vi "keccak.ip.fifo.control.export.vi"(0 "Reset":bool, 1 "TS_RESULTS.Ready":bool, 2 "TS_PARMS.Element":u64, 3 "TS_PARMS.Valid":bool, 4 "TS_DATA.Element":u64, 5 "TS_DATA.Valid":bool) -> (14 "TS_RESULTS.Element":u64, 15 "TS_RESULTS.Valid":bool, 16 "TS_PARMS.Ready":bool, 17 "TS_DATA.Ready":bool)   [LabVIEW 2021]
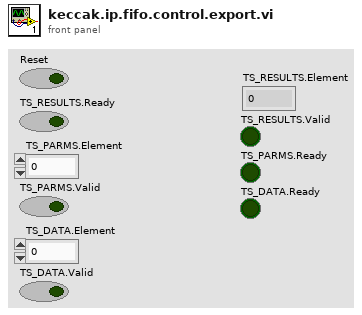
[diagram p1: front panel]
types:
  T1 = cluster{"TS_RESULTS.Ready":bool, "TS_PARMS.Element":u64, "TS_PARMS.Valid":bool, "TS_DATA.Element":u64, "TS_DATA.Valid":bool}
  T2 = cluster{"TS_RESULTS.Element":u64, "TS_RESULTS.Valid":bool, "TS_PARMS.Ready":bool, "TS_DATA.Ready":bool}
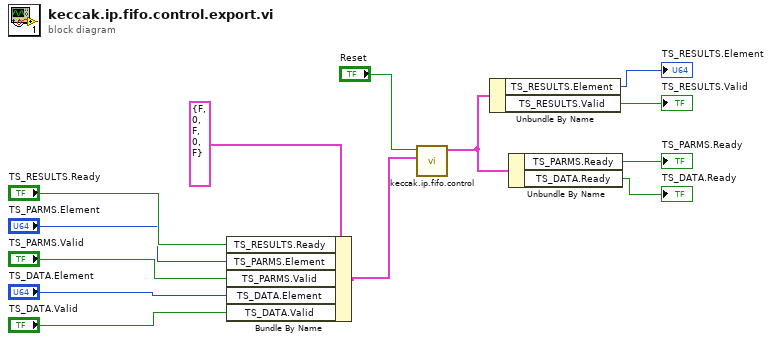
[diagram p0: block diagram]
diagram:
  n1 = Bundle By Name(cluster=T1 {"TS_RESULTS.Ready"=FALSE, "TS_PARMS.Element"=0, "TS_PARMS.Valid"=FALSE, "TS_DATA.Element"=0, "TS_DATA.Valid"=FALSE} ("FIFO.inputs"), "TS_RESULTS.Ready"="TS_RESULTS.Ready", "TS_PARMS.Element"="TS_PARMS.Element", "TS_PARMS.Valid"="TS_PARMS.Valid", "TS_DATA.Element"="TS_DATA.Element", "TS_DATA.Valid"="TS_DATA.Valid") -> (w6:T1)
  n2 = call "keccak.ip.fifo.control.vi"("FIFO.inputs"=w6, "Reset"="Reset") -> ("FIFO.outputs"=w12:T2)  [unwired: 9 in]
  n3 = Unbundle By Name(w12) -> ("TS_RESULTS.Element"=→"TS_RESULTS.Element":u64, "TS_RESULTS.Valid"=→"TS_RESULTS.Valid":bool)
  n4 = Unbundle By Name(w12) -> ("TS_PARMS.Ready"=→"TS_PARMS.Ready":bool, "TS_DATA.Ready"=→"TS_DATA.Ready":bool)
